vi "Parameters filler.vi"(8 "error in (no error)":errorcluster, 9 "FPGA Name":string, 10 "Subpanels Map":map{string, refnum<vi>}(c390), 11 "Parameters Map":map{string, string[]}(c390)) -> (0 "error out":errorcluster)   [LabVIEW 2020, in "Scheduler.lvlib"]
uses:
  Scheduler.lvlib
  Ancestor/Ancestor/Ancestor.lvclass/Ancestor.ctl
  Support VIs/Generate Error.vi
  FGV/Error Memory/Get Error Description.vi
  Support VIs/Get PC name.vi
  Ancestor/Ancestor/Read ID.vi
  Support VIs/Get Class Name.vi
  <vilib>/Utility/error.llb/Clear Errors.vi
  FGV/Error Memory/Error Memory Core.vi
  <vilib>/AdvancedString/Delimited String to 1D String Array.vi
  Support VIs/Circus Root Path.vi
  FGV/Error Memory/Error Crt Lvl checker.vi
  FGV/Error Memory/Error Memory Core.vi/40c8088d-b597-4017-91af-faa98e00292e.vi
  FGV/Error Memory/Error Memory Core.vi/d4a3ab98-063c-4e44-b43d-fbdcfe6c2be2.vi
  Add RUN Window.vi
  Support VIs/Global Memory.vi
  <vilib>/Utility/LVClass/Get LV Class Name.vi
  Support VIs/Is in Packed Library.vi
  Support VIs/TALOS Root path.vi
  Support VIs/Read CSV worksheet.vi
  Support VIs/Global Constants.vi
  <vilib>/Utility/error.llb/General Error Handler.vi
  Support VIs/Error Log.vi
  Ancestor/Ancestor/Ancestor.lvclass
  <vilib>/Comparison/Equal/Equal Functor/Equal Functor.lvclass
  TALOS.lvlib
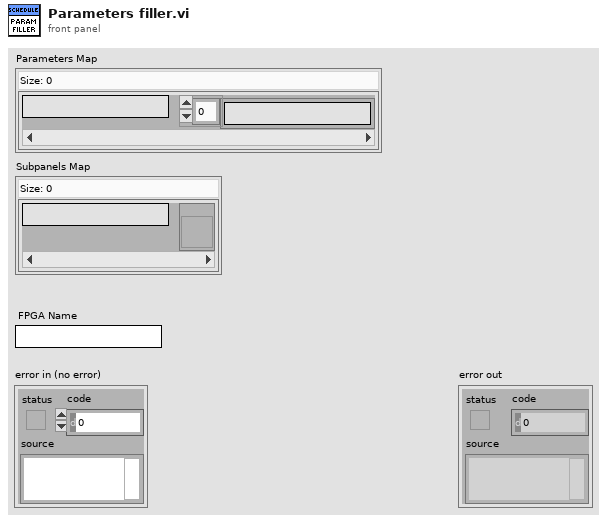
[diagram p1: front panel]
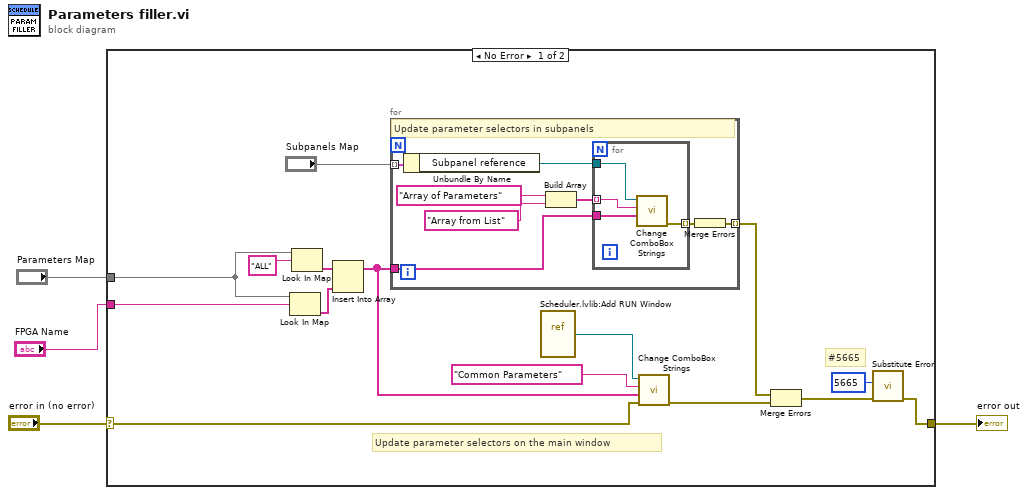
[diagram p0: block diagram]
diagram:
  n1 = case shown="No Error" "error in (no error)" {
    selector: "error in (no error)" -> [w16 w32]
    tunnel: [w18 w32] -> w3
    tunnel: "Parameters Map" -> [w8 _]
    tunnel: "FPGA Name" -> [w7 _]
    frame No Error {
      # "Update parameter selectors on the main window"
      # "#5665"
      n2 = Look In Map(map=w8, key=w7) -> (value=w12:string[])  [unwired: 1 in, 1 out]
      n3 = Look In Map(map=w8, key="ALL") -> (value=w13:string[])  [unwired: 1 in, 1 out]
      n4 = Insert Into Array(array=w13, new element=w12) -> (w11:string[])  [unwired: 1 in]
      n5 = for {
        tunnel: w11 -> [w27]
        tunnel: [w22] -> w10 mode=indexing
        tunnel: "Subpanels Map" -> [w21] mode=indexing
        # "Update parameter selectors in subpanels"
        n6 = Unbundle By Name(w21) -> ("Subpanel reference"=w20:refnum<vi>)
        n7 = Build Array("Array of Parameters" ("Control Name"), "Array from List" ("Control Name")) -> (w23:string[])
        n8 = for {
          tunnel: w27 -> [w31]
          tunnel: w23 -> [w30] mode=indexing
          tunnel: [w29] -> w26 mode=indexing
          tunnel: w20 -> [w28]
          n9 = call "Change ComboBox Strings.vi"("Parameters"=w31, "Control Name"=w30, "VI reference in"=w28) -> ("error out"=w29:errorcluster)  [unwired: 5 in, 1 out]
        }
        n10 = Merge Errors(w26) -> (w22:errorcluster)
      }
      n11 = vi-ref "Scheduler.lvlib:Add RUN Window.vi"() -> (w5:refnum<vi>)
      n12 = call "Change ComboBox Strings.vi"("error in"=w16, "Parameters"=w11, "Control Name"="Common Parameters", "VI reference in"=w5) -> ("error out"=w9:errorcluster)  [unwired: 4 in, 1 out]
      n13 = Merge Errors(w10, w9) -> (w19:errorcluster)
      n14 = call "Substitute Error.vi"("error in (no error)"=w19, "Error Code"=5665) -> ("error out"=w18:errorcluster)  [unwired: 9 in]
    }
    frame Error {
    }
  }
  "error out" <- w3
